vi "位置初始化判断.vi"(6 "位置初始化":dbl, 10 "是否后退":bool) -> (2 "位置判断":dbl)   [LabVIEW 2015]
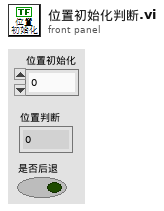
[diagram p1: front panel]
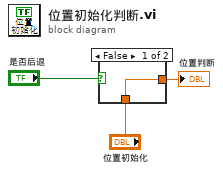
[diagram p0: block diagram]
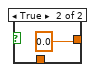
[diagram p2: hidden frame]
diagram:
  n1 = case shown="False" "是否后退" {
    tunnel: [w4 0.0 ("x")] -> w2
    tunnel: "位置初始化" -> [w4 _]
    frame False {
    }
    frame True {
    }
  }
  "位置判断" <- w2
